vi "FTW-Message-Core-Receive.vi"(0 "Incoming Message":refnum<class "FTW-Message.lvclass">, 2 "Expected Message Type":refnum<class "FTW-Message.lvclass">, 11 "error in":errorcluster) -> (4 "Constructed Message Type":refnum<class "FTW-Message.lvclass">, 6 "Message":string, 15 "error out":errorcluster)   [LabVIEW 2013, in "FTW-Message.lvclass"]
uses:
  FTW-Message.lvclass
  FTW-Message.lvclass/FTW-Message.ctl
panel:
  # "Inputs"
  # "Outputs"
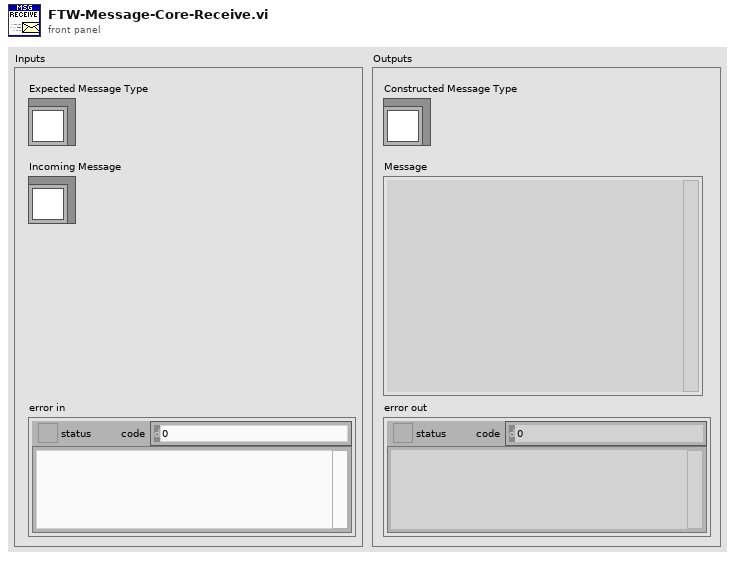
[diagram p1: front panel]
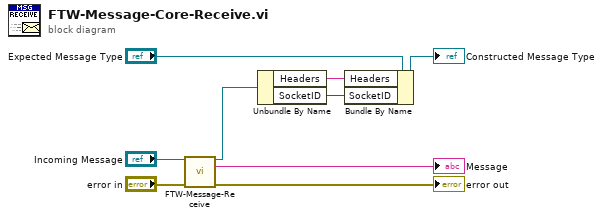
[diagram p0: block diagram]
diagram:
  n1 = call "FTW-Message-Receive.vi"("FTW Incoming Message"="Incoming Message", "error in"="error in") -> ("FTW Incoming Message out"=w4:refnum<class "FTW-Message.lvclass">, "Message"=→"Message":string, "error out"=→"error out":errorcluster)  [unwired: 11 in]
  n2 = Unbundle By Name(w4) -> ("Headers"=w7:string, "SocketID"=w6:i64)
  n3 = Bundle By Name(cluster="Expected Message Type", "Headers"=w7, "SocketID"=w6) -> (→"Constructed Message Type":refnum<class "FTW-Message.lvclass">)
